vi "Wrap Update Loaded Plugins.vi"(8 "error in (no error)":errorcluster, 11 "CIF_UI in":refnum<class "CIF_UI.lvclass">) -> (0 "error out":errorcluster, 3 "CIF_UI out":refnum<class "CIF_UI.lvclass">)   [LabVIEW 2021, in "CIF_UI.lvclass"]
uses:
  CIF_UI.lvclass
  CIF_UI.lvclass/CIF_UI.ctl
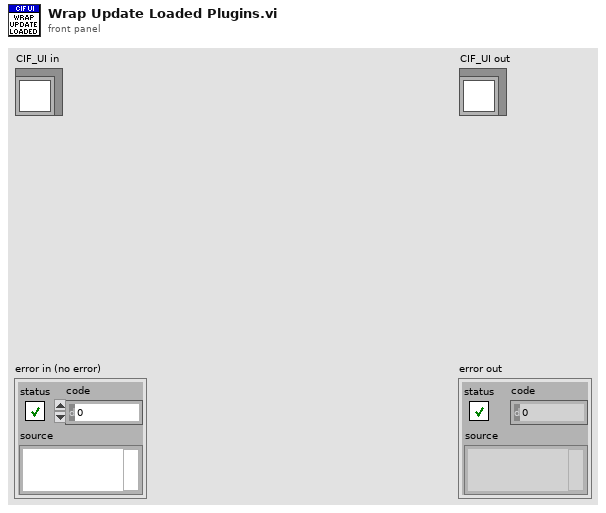
[diagram p1: front panel]
types:
  T1 = typedef "CIF_UI.lvclass/Plugin Summary.ctl" = cluster{"Name":string, "Type":string, "grpc_port":i32, "Version":T2}
  T2 = typedef "CIF_UI.lvclass/Version.ctl" = cluster{"Major":i32, "Minor":i32, "Fix":i32}
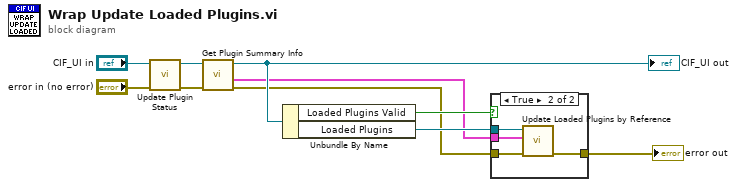
[diagram p0: block diagram]
diagram:
  n1 = call "Update Plugin Status.vi"("error in (no error)"="error in (no error)", "CIF_UI in"="CIF_UI in") -> ("error out"=w5:errorcluster, "CIF_UI out"=w6:refnum<class "CIF_UI.lvclass">)  [unwired: 8 in]
  n2 = call "Get Plugin Summary Info.vi"("error in (no error)"=w5, "CIF_UI in"=w6) -> ("error out"=w3:errorcluster, "Plugin Summary Info"=w2:T1[], "CIF_UI out"=w4:refnum<class "CIF_UI.lvclass">)  [unwired: 7 in]
  "CIF_UI out" <- w4
  n3 = Unbundle By Name(w4) -> ("Loaded Plugins Valid"=w8:bool, "Loaded Plugins"=w7:refnum<vi>)
  n4 = case shown="True" w8 {
    tunnel: w7 -> [_ w15]
    tunnel: w3 -> [w11 w14]
    tunnel: [w11 w13] -> w1
    tunnel: w2 -> [_ w12]
    frame False {
    }
    frame True {
      n5 = call "Update Loaded Plugins by Reference.vi"("error in (no error)"=w14, "Plugin Summary Info"=w12, "Loaded Plugins ref in"=w15) -> ("error out"=w13:errorcluster)  [unwired: 7 in, 1 out]
    }
  }
  "error out" <- w1
